vi "WFS_Thorlabs_FGV.vi"(6 "Zernike fit?":bool, 7 "State":T2, 8 "error in":errorcluster, 9 "WF and Zernike fit config":T3={"Limit meas. to pupil"=0, "Cancel WF tilt"=enum."No", "Zern. order max."=5, "wavelength, um"=0.633} {"wavelength, um" format="%.3f"; "Limit meas. to pupil" items=["Yes"=1, "No"=0]}, 10 "WFS cam & pupil config":T4={"Trigger Mode"=enum."Continuous", "Auto exposure"=FALSE, "Exposure time (ms)"=0.07936666666666667, "Master gain"=1.0, "Cam img size"=1, "Pupil diam X (mm)"=4.5, "Pupil diam Y (mm)"=4.5} {"Cam img size" items=["1280x1024 = 5.95x4.76mm", "1024x1024 = 4.76x4.76mm", "768x768 = 3.57x3.57mm", "512x512 = 2.38x2.38mm", "320x320 = 1.49x1.49mm"]; "Exposure time (ms)" min=0.0793667 max=66.6148 step=0.0554 format="%#.6f"}) -> (0 "error out":errorcluster, 1 "WF data Out":T1, 2 "WFS connected":bool)   [LabVIEW 2016]
uses:
  Type definitions/WFS cam and pupil config.ctl
  Type definitions/WFS wavefront and Zernike fit.ctl
  Type definitions/WFS wavefront data.ctl
  Type definitions/State control in WFS_Thorlabs_FGV.ctl
  <vilib>/Analysis/5stat.llb/RMS (DBL).vi
  <vilib>/Analysis/baseanly.llb/Mean (DBL).vi
  <vilib>/Analysis/NI_AALBase.lvlib
  <vilib>/Analysis/NI_AALPro.lvlib
panel:
  out "Rad. of curvature (mm)":dbl
  out "Light power":string
  out "Ambient light":string
  out "spots_y":i32
  out "spots_x":i32
  out "Exp Time Incr":dbl=0.0554 caption="Exposure Time Incr"
  out "Exp time Max, ms":dbl=66.6147666666 caption="Exposure Time Max"
  out "Exp time Min, ms":dbl=0.07936666666666665 caption="Exposure Time Min"
  out "InstName":string caption="Instrument Name"
  # "For Shack-Hartmann sensor models:\nThorlabs WFS-150, WFS-300, WFS-20"
  # "Shack-Hartmann wavefront sensor config"
  # "All units are lambda (wavelength)"
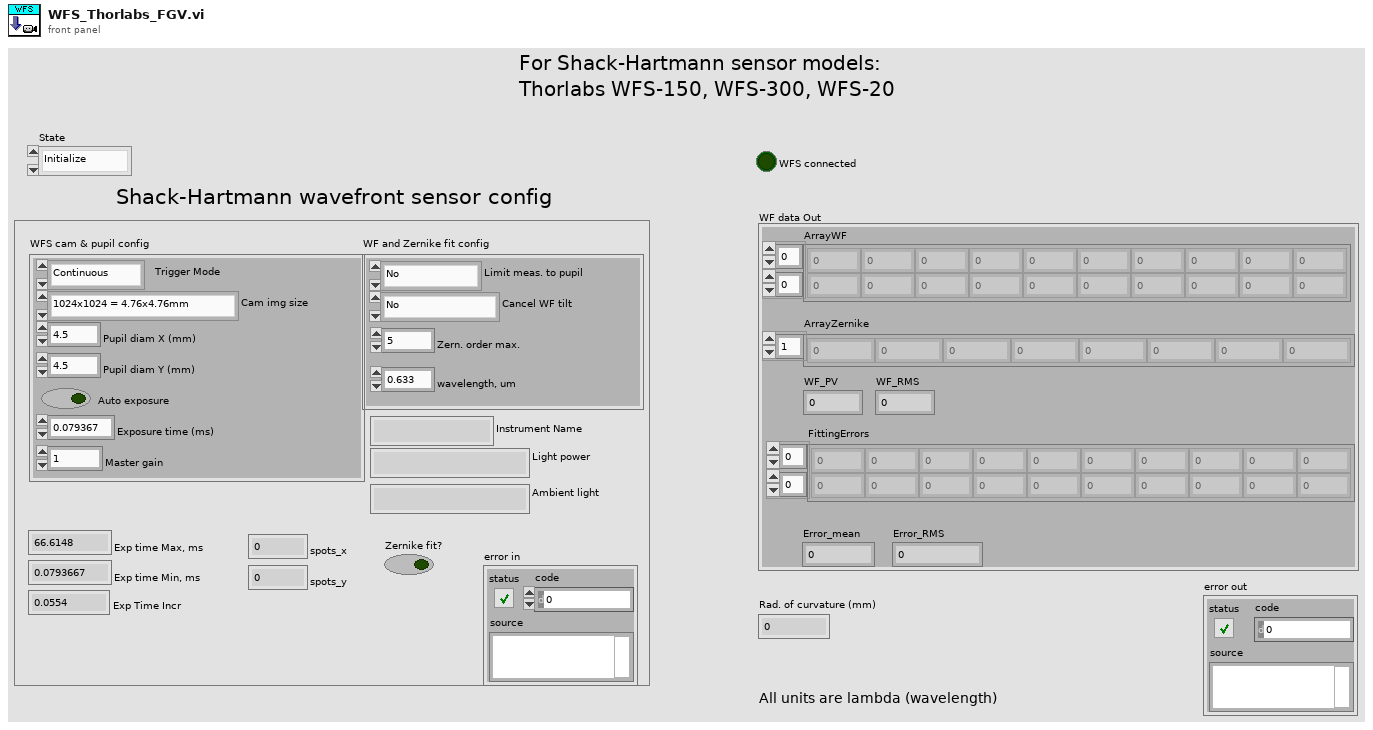
[diagram p1: front panel]
types:
  T1 = typedef "WFS wavefront data.ctl" = cluster{"ArrayWF":sgl[][], "ArrayZernike":sgl[], "WF_PV":dbl, "WF_RMS":dbl, "FittingErrors":dbl[][], "Error_mean":dbl, "Error_RMS":dbl}
  T2 = typedef "State control in WFS_Thorlabs_FGV.ctl" = enum16{"Initialize", "Configure", "Measure", "Exit"}
  T3 = typedef "WFS wavefront and Zernike fit.ctl" = cluster{"Limit meas. to pupil":i32, "Cancel WF tilt":enum16{"No", "Yes"}, "Zern. order max.":i32, "wavelength, um":dbl}
  T4 = typedef "WFS cam and pupil config.ctl" = cluster{"Trigger Mode":enum16{"Continuous", "Slope H->L", "Slope L->H", "Software"}, "Auto exposure":bool, "Exposure time (ms)":dbl, "Master gain":dbl, "Cam img size":i32, "Pupil diam X (mm)":dbl, "Pupil diam Y (mm)":dbl}
  T5 = enum16{"Continuous", "Slope H->L", "Slope L->H", "Software"}
  T6 = cluster{"ArrayWF":dbl[][], "ArrayZernike":dbl[], "WF_PV":dbl, "WF_RMS":dbl, "FittingErrors":dbl[][], "Error_mean":dbl, "Error_RMS":dbl}
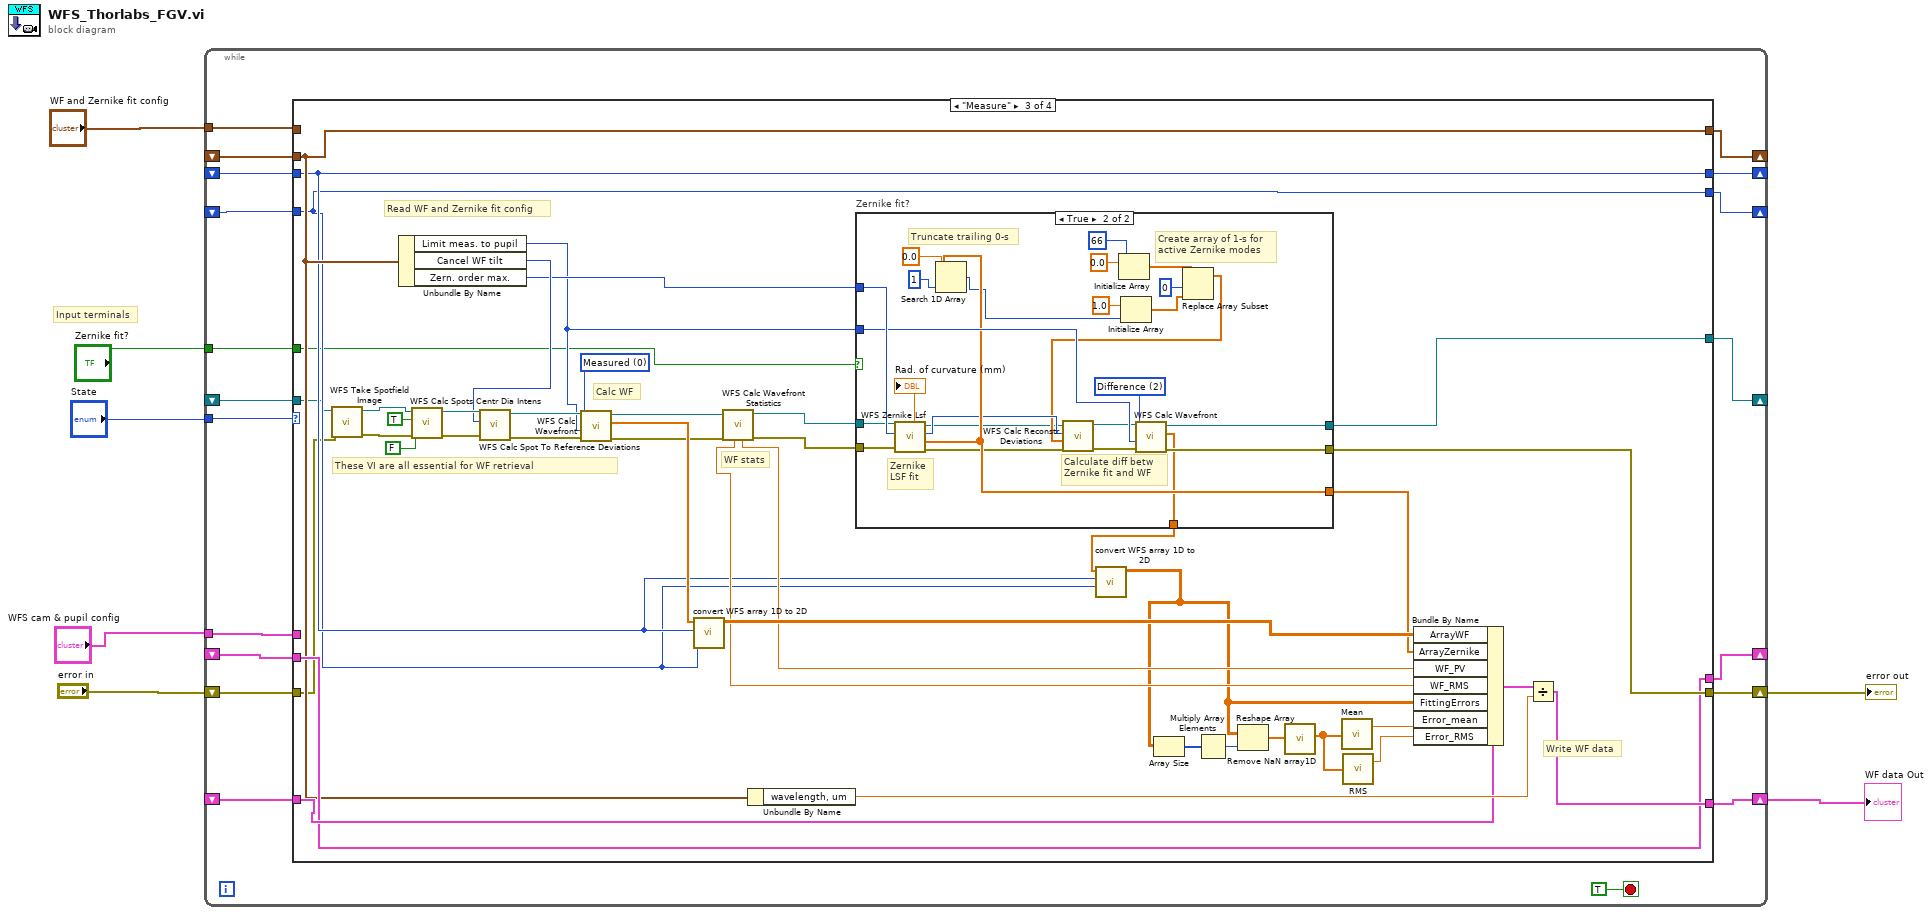
[diagram p0: block diagram]
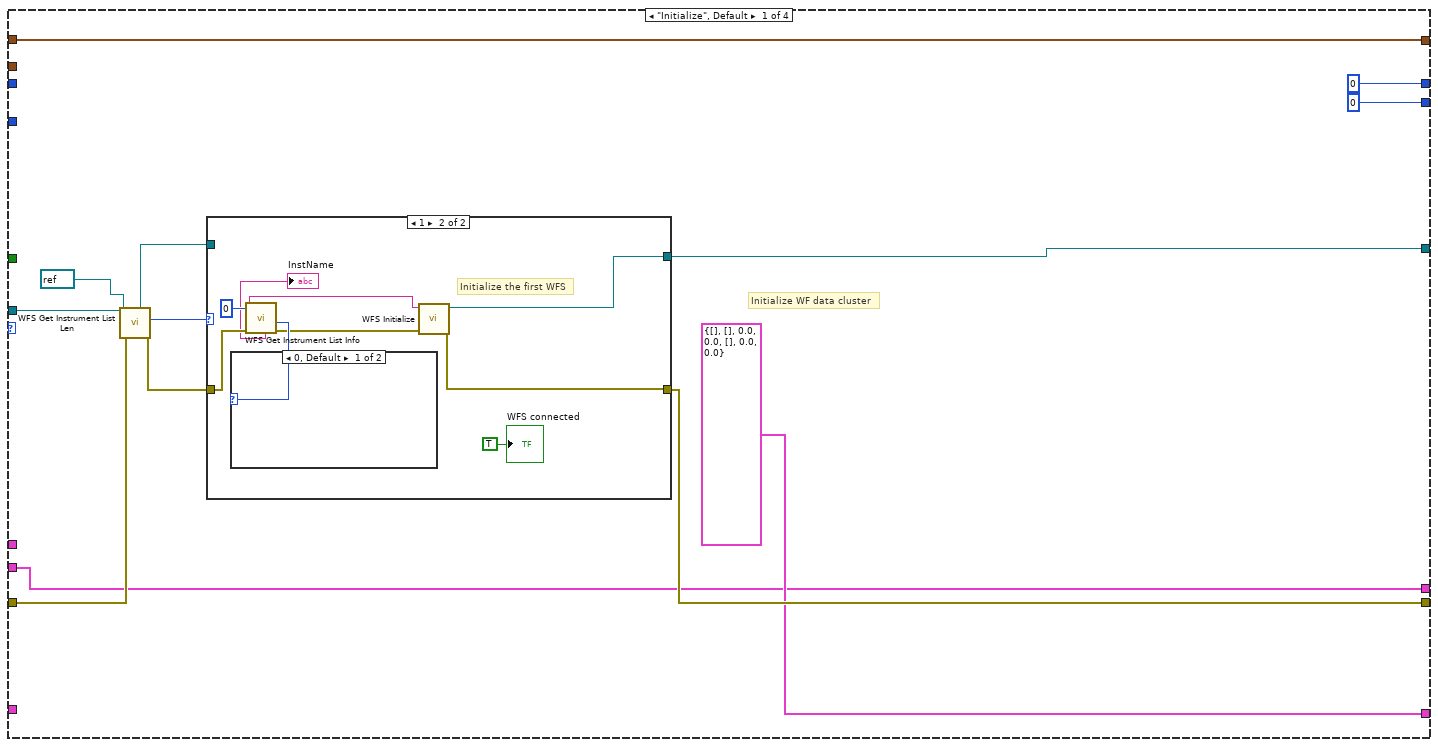
[diagram p2: hidden frame]
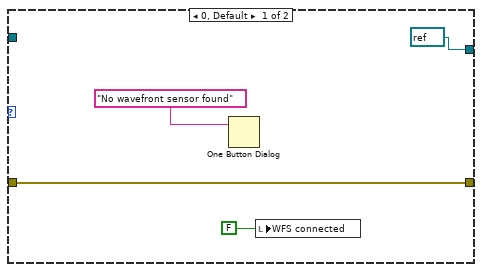
[diagram p3: hidden frame]
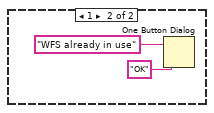
[diagram p4: hidden frame]
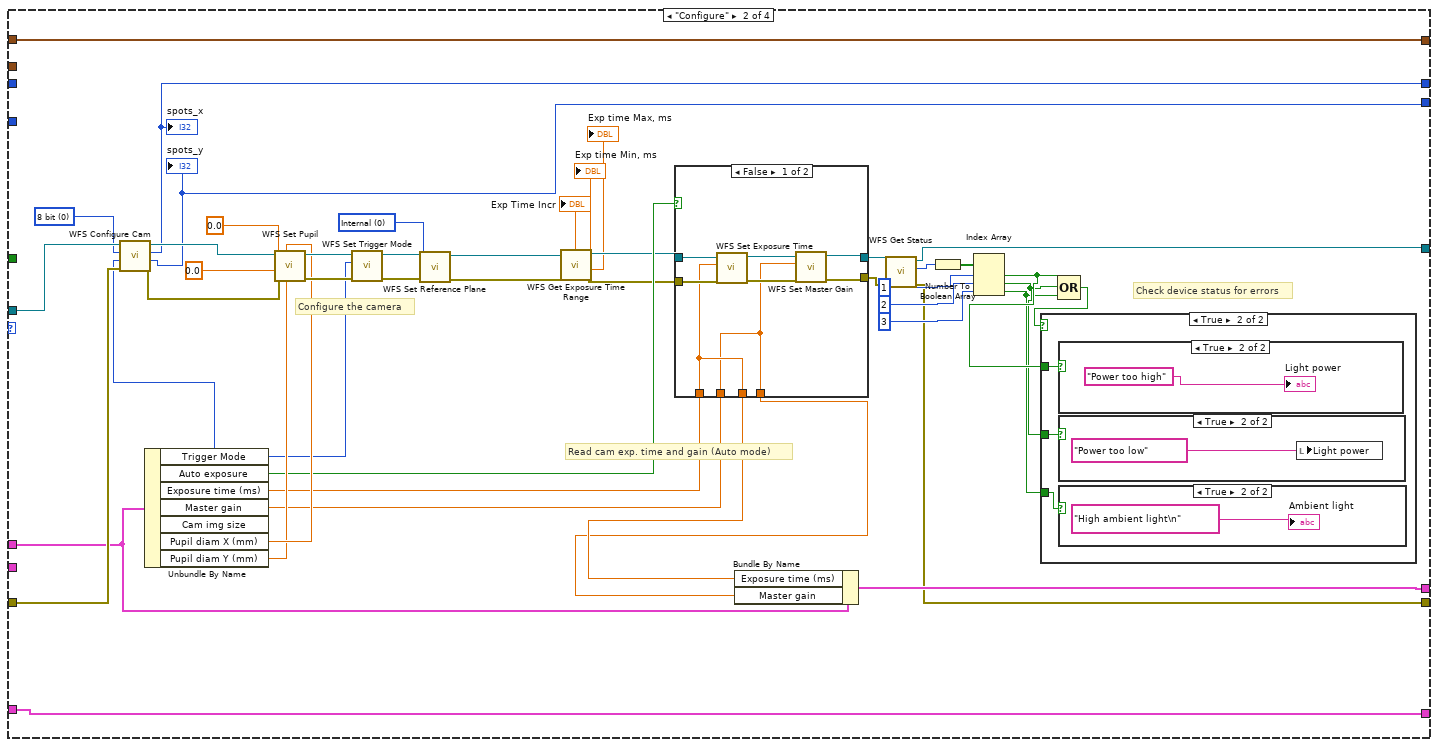
[diagram p5: hidden frame]
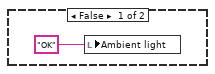
[diagram p7: hidden frame]
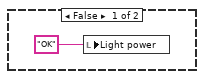
[diagram p8: hidden frame]
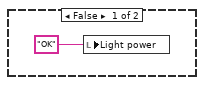
[diagram p9: hidden frame]
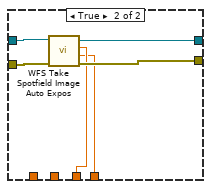
[diagram p10: hidden frame]
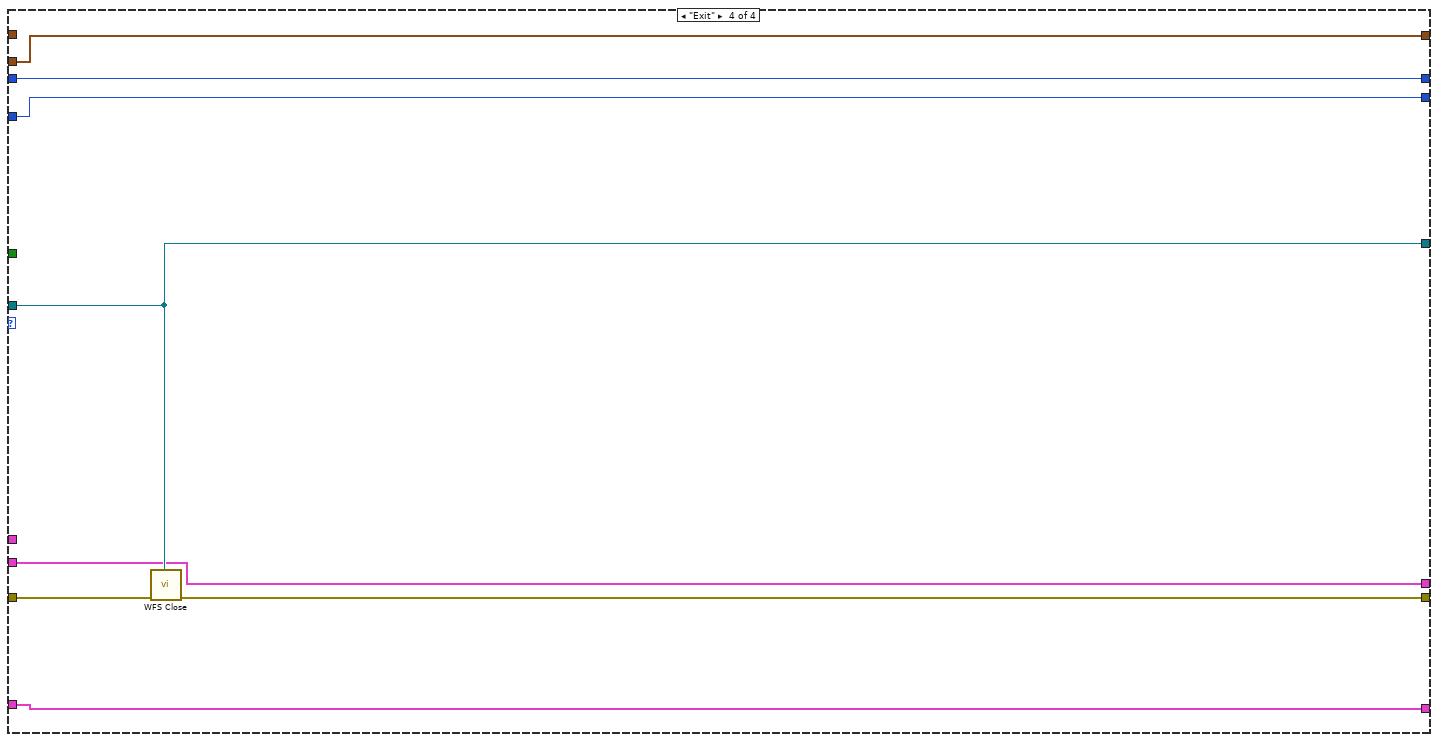
[diagram p12: hidden frame]
diagram:
  # "Input terminals"
  n1 = while {
    shift-right: [w25] -> w3
    shift-left: "error in" -> [w26]
    shift-right: [w24] -> _
    shift-left: _ -> [w23]
    tunnel: "State" -> [w22]
    shift-right: [w18] -> w2
    shift-left: _ -> [w19]
    tunnel: "WFS cam & pupil config" -> [w21]
    shift-right: [w16] -> _
    shift-left: _ -> [w15]
    tunnel: "WF and Zernike fit config" -> [w20]
    shift-right: [w14] -> _
    shift-left: _ -> [w13]
    shift-right: [w11] -> _
    shift-left: _ -> [w9]
    shift-right: [w12] -> _
    shift-left: _ -> [w10]
    tunnel: "Zernike fit?" -> [w8]
    stop <- TRUE stop-if-true
    n2 = case shown="\"Measure\"" w22 {
      tunnel: w26 -> [w38 w99 w133 w199]
      tunnel: [w34 w60 w139 w198] -> w25
      tunnel: [w33 w61 w140 w200] -> w24
      tunnel: w23 -> [w32 w100 w131 w200]
      tunnel: w21 -> [_ w81 _ _]
      tunnel: [w29 w80 w137 w196] -> w16
      tunnel: w20 -> [w31 w72 _ _]
      tunnel: [w31 w72 w136 w195] -> w14
      tunnel: w19 -> [_ w71 w142 w197]
      tunnel: [T1 {"ArrayWF"=[], "ArrayZernike"=[], "WF_PV"=0.0, "WF_RMS"=0.0, "FittingErrors"=[], "Error_mean"=0.0, "Error_RMS"=0.0} ("WF data Ini") w71 w141 w197] -> w18
      tunnel: w15 -> [w29 _ w137 w196]
      tunnel: w13 -> [_ _ w136 w195]
      tunnel: [0 ("Spots Y") w57 w134 w193] -> w11
      tunnel: [0 ("Spots X") w56 w135 w194] -> w12
      tunnel: w10 -> [_ _ w135 w194]
      tunnel: w9 -> [_ _ w134 w193]
      tunnel: w8 -> [_ _ w124 _]
      frame "Initialize", Default {
        # "Initialize WF data cluster"
        n3 = call "WFS Get Instrument List Len.vi"("error in (no error)"=w38, "instrument handle"=refnum<visa-resource-name> refnum) -> ("error out"=w35:errorcluster, "Instrument Count"=w36:i32)  [unwired: 7 in, 1 out]
        n4 = case shown="1" w36 {
          tunnel: [w41 w46] -> w34
          tunnel: w35 -> [w41 w50]
          tunnel: [refnum<visa-resource-name> refnum ("instrument handle out") w47] -> w33
          tunnel: w32 -> [_ _]
          frame 0, Default {
            n5 = One Button Dialog(message="No wavefront sensor found") -> ()  [unwired: 1 in, 1 out]
            n6 = local write "WFS connected"(FALSE ("WFS connected")) -> ()
          }
          frame 1 {
            # "Initialize the first WFS"
            n7 = call "WFS Get Instrument List Info.vi"("error in (no error)"=w50, "Instrument List Index"=0) -> ("error out"=w48:errorcluster, "In Use"=w49:i32, "Instrument Name"=→"InstName":string, "Resource Name"=w45:string)  [unwired: 3 in, 3 out]
            n8 = case shown="0, Default" w49 {
              frame 0, Default {
              }
              frame 1 {
                n9 = One Button Dialog(message="WFS already in use", button name ("OK")="OK") -> ()  [unwired: 1 out]
              }
            }
            n10 = call "WFS Initialize.vi"("error in (no error)"=w48, "resource name"=w45) -> ("error out"=w46:errorcluster, "instrument handle out"=w47:refnum<visa-resource-name>)  [unwired: 8 in]
            "WFS connected" <- TRUE ("WFS connected")
          }
        }
      }
      frame "Configure" {
        w89 = 0 items=["Internal", "User"] ("Reference Index (Internal)")
        w92 = 0 items=["16 bit"=1, "8 bit"=0] ("Pixel Format (8 bit)")
        # "Check device status for errors"
        # "Read cam exp. time and gain (Auto mode)"
        # "Configure the camera"
        n11 = Unbundle By Name(w81) -> ("Trigger Mode"=w85:T5, "Auto exposure"=w84:bool, "Exposure time (ms)"=w83:dbl, "Master gain"=w82:dbl, "Cam img size"=w88:i32, "Pupil diam X (mm)"=w87:dbl, "Pupil diam Y (mm)"=w86:dbl)
        n12 = call "WFS Configure Cam.vi"("error in (no error)"=w99, "Cam Resol. Index (1280x1024      640x480      1440x1080)"=w88, "Pixel Format (8 bit)"=w92, "instrument handle"=w100) -> ("error out"=w98:errorcluster, "Spots Y"=w57:i32, "Spots X"=w56:i32, "instrument handle out"=w97:refnum<visa-resource-name>)  [unwired: 4 in]
        "spots_y" <- w57
        "spots_x" <- w56
        n13 = call "WFS Set Pupil.vi"("Pupil Diameter Y mm"=w86, "Pupil Diameter X mm"=w87, "error in (no error)"=w98, "Pupil Center Y mm"=0.0, "Pupil Center X mm"=0.0, "instrument handle"=w97) -> ("error out"=w95:errorcluster, "instrument handle out"=w96:refnum<visa-resource-name>)  [unwired: 4 in]
        n14 = call "WFS Set Trigger Mode.vi"("error in (no error)"=w95, "Trigger Mode"=w85, "instrument handle"=w96) -> ("error out"=w90:errorcluster, "instrument handle out"=w91:refnum<visa-resource-name>)  [unwired: 7 in]
        n15 = call "WFS Set Reference Plane.vi"("error in (no error)"=w90, "Reference Index (Internal)"=w89, "instrument handle"=w91) -> ("error out"=w54:errorcluster, "instrument handle out"=w55:refnum<visa-resource-name>)  [unwired: 7 in]
        n16 = call "WFS Get Exposure Time Range.vi"("error in (no error)"=w54, "instrument handle"=w55) -> ("error out"=w76:errorcluster, "Exposure Time Max"=→"Exp time Max, ms":dbl, "Exposure Time Min"=→"Exp time Min, ms":dbl, "instrument handle out"=w77:refnum<visa-resource-name>, "Exposure Time Incr"=→"Exp Time Incr":dbl)  [unwired: 5 in]
        n17 = case shown="False" w84 {
          tunnel: [w115 w123] -> w63
          tunnel: [w114 w122] -> w62
          tunnel: w76 -> [w113 w120]
          tunnel: w77 -> [w112 w121]
          tunnel: w83 -> [w111 _]
          tunnel: w82 -> [w110 _]
          tunnel: [w111 w119] -> w79
          tunnel: [w110 w118] -> w78
          frame False {
            n18 = call "WFS Set Exposure Time.vi"("error in (no error)"=w113, "Exposure Time Set"=w111, "instrument handle"=w112) -> ("error out"=w117:errorcluster, "instrument handle out"=w116:refnum<visa-resource-name>)  [unwired: 6 in, 1 out]
            n19 = call "WFS Set Master Gain.vi"("error in (no error)"=w117, "Master Gain Set"=w110, "instrument handle"=w116) -> ("error out"=w114:errorcluster, "instrument handle out"=w115:refnum<visa-resource-name>)  [unwired: 6 in, 1 out]
          }
          frame True {
            n20 = call "WFS Take Spotfield Image Auto Expos.vi"("error in (no error)"=w120, "instrument handle"=w121) -> ("error out"=w122:errorcluster, "Master Gain Act"=w118:dbl, "Exposure Time Act"=w119:dbl, "instrument handle out"=w123:refnum<visa-resource-name>)  [unwired: 6 in]
          }
        }
        n21 = Bundle By Name(cluster=w81, "Exposure time (ms)"=w79, "Master gain"=w78) -> (w80:T4)
        n22 = call "WFS Get Status.vi"("error in (no error)"=w62, "instrument handle"=w63) -> ("error out"=w60:errorcluster, "Device Status"=w59:i32, "instrument handle out"=w61:refnum<visa-resource-name>)  [unwired: 7 in]
        n23 = Number To Boolean Array(number=w59) -> (Boolean array=w58:bool[])
        n24 = Index Array(array=w58, index #1=1 ("index"), index #2=2 ("index"), index #3=3 ("index")) -> (element #1=w66:bool, element #2=w65:bool, element #3=w64:bool)
        n25 = Compound Arithmetic op=OR(w66, w65, w64) -> (w67:bool)
        n26 = case shown="True" w67 {
          tunnel: w66 -> [_ w103]
          tunnel: w65 -> [_ w102]
          tunnel: w64 -> [_ w101]
          frame False {
          }
          frame True {
            n27 = case shown="True" w103 {
              frame False {
                n28 = local write "Light power"("OK" ("Device Status")) -> ()
              }
              frame True {
                "Light power" <- "Power too high"
              }
            }
            n29 = case shown="True" w102 {
              frame False {
                n30 = local write "Light power"("OK" ("Device Status")) -> ()
              }
              frame True {
                n31 = local write "Light power"("Power too low") -> ()
              }
            }
            n32 = case shown="True" w101 {
              frame False {
                n33 = local write "Ambient light"("OK" ("Device Status 2")) -> ()
              }
              frame True {
                "Ambient light" <- "High ambient light\n"
              }
            }
          }
        }
      }
      frame "Measure" {
        w157 = 0 items=["Measured", "Reconstructed", "Difference"] ("Wavefront Type (Measured)")
        # "WF stats"
        # "Write WF data"
        # "Calc WF"
        # "Read WF and Zernike fit config"
        # "These VI are all essential for WF retrieval"
        n34 = call "WFS Take Spotfield Image.vi"("error in (no error)"=w133, "instrument handle"=w131) -> ("error out"=w132:errorcluster, "instrument handle out"=w130:refnum<visa-resource-name>)  [unwired: 8 in]
        n35 = Unbundle By Name(w136) -> ("Limit meas. to pupil"=w155:i32, "Cancel WF tilt"=w158:enum16{"No", "Yes"}, "Zern. order max."=w156:i32)
        n36 = call "WFS Calc Spots Centr Dia Intens.vi"("error in (no error)"=w132, "Calculate Diameters (Off)"=FALSE, "Dynamic Noise Cut (On)"=TRUE, "instrument handle"=w130) -> ("error out"=w161:errorcluster, "instrument handle out"=w162:refnum<visa-resource-name>)  [unwired: 6 in]
        n37 = call "WFS Calc Spot To Reference Deviations.vi"("error in (no error)"=w161, "Cancel Wavefront Tilt (No)"=w158, "instrument handle"=w162) -> ("error out"=w160:errorcluster, "instrument handle out"=w159:refnum<visa-resource-name>)  [unwired: 7 in]
        n38 = call "WFS Calc Wavefront.vi"("error in (no error)"=w160, "Limit to Pupil (No)"=w155, "Wavefront Type (Measured)"=w157, "instrument handle"=w159) -> ("error out"=w126:errorcluster, "Array Wavefront"=w165:sgl[], "instrument handle out"=w128:refnum<visa-resource-name>)  [unwired: 5 in]
        n39 = call "convert WFS array 1D to 2D.vi"("spots_y"=w134, "spots_x"=w135, "WF 1D input"=w165) -> ("FW 2D output"=w152:sgl[][])  [unwired: 8 in]
        n40 = call "WFS Calc Wavefront Statistics.vi"("error in (no error)"=w126, "instrument handle"=w128) -> ("error out"=w125:errorcluster, "instrument handle out"=w127:refnum<visa-resource-name>, "Diff"=w150:dbl, "RMS"=w149:dbl)  [unwired: 2 in, 4 out]
        n41 = Unbundle By Name(w136) -> ("wavelength, um"=w153:dbl)
        n42 = case "Zernike fit?" shown="True" w124 {
          tunnel: w156 -> [_ w192]
          tunnel: w155 -> [_ w191]
          tunnel: [_ w190] -> w151
          tunnel: [w167 w189] -> w140
          tunnel: [w166 w188] -> w139
          tunnel: [_ w172] -> w129
          tunnel: w127 -> [w167 w171]
          tunnel: w125 -> [w166 w170]
          frame False {
          }
          frame True {
            w183 = 2 items=["Measured", "Reconstructed", "Difference"] ("Wavefront Type (Measured)")
            # "Create array of 1-s for \nactive Zernike modes"
            # "Truncate trailing 0-s"
            # "Calculate diff betw \nZernike fit and WF"
            # "Zernike \nLSF fit"
            n43 = call "WFS Zernike Lsf.vi"("error in (no error)"=w170, "Zernike Orders In"=w192, "instrument handle"=w171) -> ("error out"=w168:errorcluster, "Array Zernike um"=w190:sgl[], "Zernike Orders Out"=w186:i32, "instrument handle out"=w169:refnum<visa-resource-name>, "RoC mm"=→"Rad. of curvature (mm)":dbl)  [unwired: 3 in, 1 out]
            n44 = Search 1D Array(1D array=w190, element=sgl 0.0, start index (0)=1) -> (index of element=w176:i32)
            n45 = Initialize Array(0.0 ("element"), 66 ("dimension size")) -> (w178:dbl[])
            n46 = Initialize Array(1.0 ("element"), w176) -> (w174:dbl[])
            n47 = Replace Array Subset(array=w178, new element=w174, index=0) -> (w173:dbl[])
            n48 = call "WFS Calc Reconstr Deviations.vi"("error in (no error)"=w168, "Array Zernike Reconstruct"=w173, "Zernike Orders"=w186, "instrument handle"=w169) -> ("error out"=w185:errorcluster, "instrument handle out"=w184:refnum<visa-resource-name>)  [unwired: 4 in, 2 out]
            n49 = call "WFS Calc Wavefront.vi"("error in (no error)"=w185, "Limit to Pupil (No)"=w191, "Wavefront Type (Measured)"=w183, "instrument handle"=w184) -> ("error out"=w188:errorcluster, "Array Wavefront"=w172:sgl[], "instrument handle out"=w189:refnum<visa-resource-name>)  [unwired: 5 in]
          }
        }
        n50 = call "convert WFS array 1D to 2D.vi"("spots_y"=w134, "spots_x"=w135, "WF 1D input"=w129) -> ("FW 2D output"=w138:sgl[][])  [unwired: 8 in]
        n51 = Array Size(array=w138) -> (size(s)=w147:i32[])
        n52 = Multiply Array Elements(1:w147) -> (0:w148:i32)
        n53 = Reshape Array(w138, w148) -> (w144:sgl[])
        n54 = call "Remove NaN array1D.vi"("Array in"=w144) -> ("Array out"=w143:dbl[])  [unwired: 10 in]
        n55 = call-poly <vilib>:"Mean.vi"("X"=w143) -> ("mean"=w145:dbl)  [unwired: 1 out]
        n56 = call-poly <vilib>:"RMS.vi"("X"=w143) -> ("rms value"=w146:dbl)  [unwired: 1 out]
        n57 = Bundle By Name(cluster=w142, "ArrayWF"=w152, "ArrayZernike"=w151, "WF_PV"=w150, "WF_RMS"=w149, "FittingErrors"=w138, "Error_mean"=w145, "Error_RMS"=w146) -> (w154:T6)
        n58 = Divide(x=w154, y=w153) -> (x/y=w141:T6)
      }
      frame "Exit" {
        n59 = call "WFS Close.vi"("error in (no error)"=w199, "instrument handle"=w200) -> ("error out"=w198:errorcluster)  [unwired: 9 in]
      }
    }
  }
  "error out" <- w3
  "WF data Out" <- w2
